vi "Execute.vi"(8 "error in":errorcluster, 11 "Stabilize Laser in":refnum<class "Stabilize Laser.lvclass">) -> (0 "error out":errorcluster, 1 "Next Step?":bool, 2 "MSG":string, 3 "Stabilize Laser out":refnum<class "Stabilize Laser.lvclass">)   [LabVIEW 2013, in "Stabilize Laser.lvclass"]
uses:
  Stabilize Laser.lvclass
  Stabilize Laser.lvclass/Stabilize Laser.ctl
  Stability Step/Stability Step.lvclass/Stability Step.ctl
  Reusable/Sequence/STEPS/STEP.lvclass/STEP.ctl
  Read State DVR.vi
  Stability Step/Read # of Obs.vi
  Reusable/Sequence/STEPS/Read First Call.vi
  Stability Step/Read Error.vi
  Reusable/Sequence/STEPS/Write First Call.vi
  Reusable/PAS/Data/Main/Read CellData.vi
  Reusable/PAS/Data/Cell/Read houseKeeping.vi
  Data/cPAS Data.lvclass
  Reusable/PAS/Data/Cell/PAS Cell Data.lvclass
  <vilib>/Analysis/NI_AALBase.lvlib
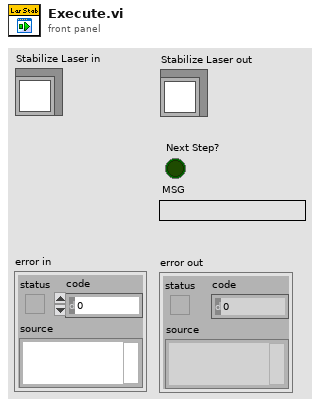
[diagram p1: front panel]
types:
  T1 = cluster{"T":sgl, "TRH":sgl, "RH":sgl, "laserRMS":sgl}
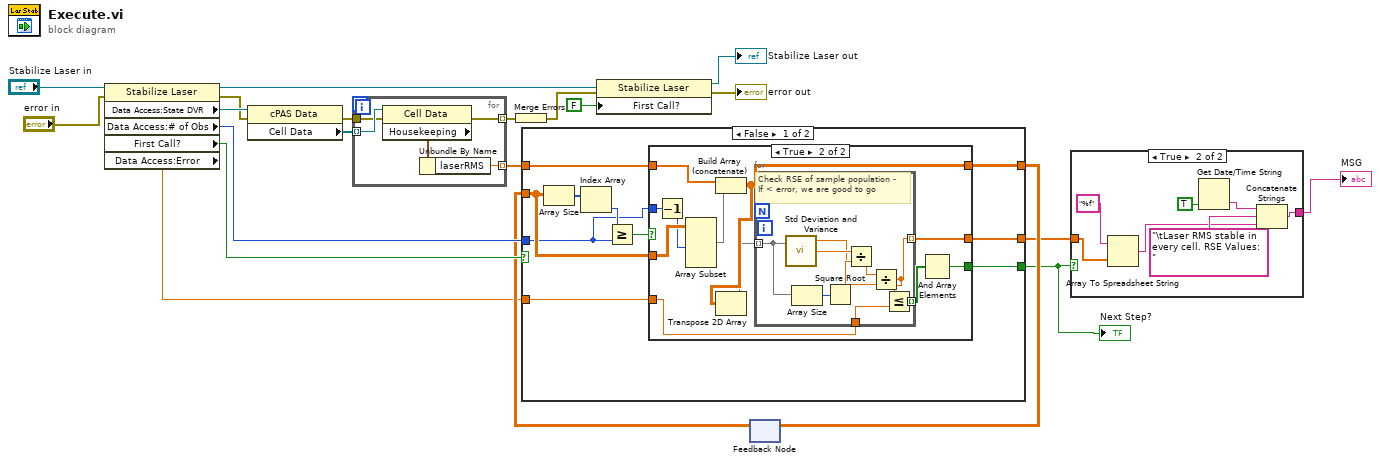
[diagram p0: block diagram]
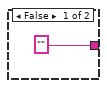
[diagram p2: hidden frame]
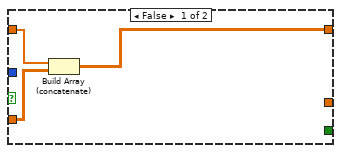
[diagram p3: hidden frame]
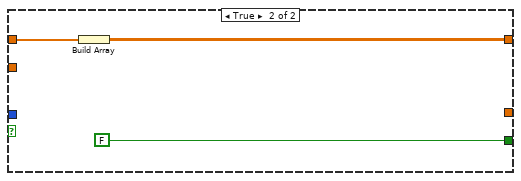
[diagram p4: hidden frame]
diagram:
  n1 = property class="Stabilize Laser"(reference="Stabilize Laser in", error in="error in") -> (reference out=w20:refnum<class "Stabilize Laser.lvclass">, error out=w3:errorcluster, "Data Access:State DVR"=w4:refnum<data-value>, "Data Access:# of Obs"=w17:u16, "First Call?"=w18:bool, "Data Access:Error"=w2:sgl)
  n2 = property class="cPAS Data"(reference=w4, error in=w3) -> (error out=w13:errorcluster, "Cell Data"=w21:refnum<class "PAS Cell Data.lvclass">[])  [unwired: 1 out]
  n3 = for {
    tunnel: w21 -> [w26] mode=indexing
    tunnel: [w24] -> w16 mode=indexing
    tunnel: w13 -> [w23]
    tunnel: [w22] -> w12 mode=indexing
    n4 = property class="Cell Data"(reference=w26, error in=w23) -> (error out=w22:errorcluster, "Housekeeping"=w25:T1)  [unwired: 1 out]
    n5 = Unbundle By Name(w25) -> ("laserRMS"=w24:sgl)
  }
  n6 = Merge Errors(w12) -> (w11:errorcluster)
  n7 = property class="Stabilize Laser"(reference=w20, error in=w11, "First Call?"=FALSE) -> (reference out=→"Stabilize Laser out":refnum<class "Stabilize Laser.lvclass">, error out=→"error out":errorcluster)
  n8 = feedback #1() -> (w14:sgl[][])  [unwired: 1 in]
  n9 = case shown="False" w18 {
    tunnel: w17 -> [w28 _]
    tunnel: w16 -> [w34 w62]
    tunnel: [w32 w61] -> w15
    tunnel: w14 -> [w33 _]
    tunnel: [w29 FALSE ("Boolean")] -> w5
    tunnel: w2 -> [w30 _]
    tunnel: [w27 _] -> w1
    frame False {
      n10 = Array Size(array=w33) -> (size(s)=w36:i32[])
      n11 = Index Array(array=w36) -> (element=w31:i32)  [unwired: 1 in]
      n12 = Greater Or Equal?(x=w31, y=w28) -> (x >= y?=w35:bool)
      n13 = case shown="True" w35 {
        tunnel: w34 -> [w39 w48]
        tunnel: w33 -> [w38 w50]
        tunnel: [w37 w44] -> w32
        tunnel: w30 -> [_ w41]
        tunnel: [_ w47] -> w29
        tunnel: w28 -> [_ w46]
        tunnel: [_ w42] -> w27
        frame False {
          n14 = Build Array (concatenate)(w39, w38) -> (w37:sgl[][])
        }
        frame True {
          n15 = Decrement(x=w46) -> (x-1=w45:u16)
          n16 = Array Subset(array=w50, length (row)=w45) -> (w49:sgl[][])  [unwired: 3 in]
          n17 = Build Array (concatenate)(w48, w49) -> (w44:sgl[][])
          n18 = Transpose 2D Array(2D array=w44) -> (transposed array=w43:sgl[][])
          n19 = for {
            tunnel: w43 -> [w59] mode=indexing
            tunnel: [w53] -> w42 mode=indexing
            tunnel: w41 -> [w52]
            tunnel: [w51] -> w40 mode=indexing
            # "Check RSE of sample population -\nIf < error, we are good to go"
            n20 = call <vilib>:"Std Deviation and Variance.vi"("X"=w59) -> ("mean"=w54:dbl, "standard deviation"=w57:dbl)  [unwired: 1 in, 1 out]
            n21 = Array Size(array=w59) -> (size(s)=w58:i32)
            n22 = Square Root(x=w58) -> (sqrt(x)=w56:dbl)
            n23 = Divide(x=w57, y=w56) -> (x/y=w55:dbl)
            n24 = Divide(x=w55, y=w54) -> (x/y=w53:dbl)
            n25 = Less Or Equal?(x=w53, y=w52) -> (x <= y?=w51:bool)
          }
          n26 = And Array Elements(Boolean array=w40) -> (logical AND=w47:bool)
        }
      }
    }
    frame True {
      n27 = Build Array(w62) -> (w61:sgl[][])
    }
  }
  "Next Step?" <- w5
  n28 = feedback-in #1(w15) -> ()
  n29 = case shown="True" w5 {
    tunnel: ["" w68] -> w6
    tunnel: w1 -> [_ w64]
    frame False {
    }
    frame True {
      n30 = Array To Spreadsheet String(array=w64, 3:"%f" ("format string")) -> (spreadsheet string=w66:string)  [unwired: 1 in]
      n31 = Get Date/Time String(want seconds? (F)=TRUE) -> (time string=w69:string)  [unwired: 2 in, 1 out]
      n32 = Concatenate Strings(w69, "\tLaser RMS stable in every cell. RSE Values: " ("string"), w66) -> (w68:string)
    }
  }
  "MSG" <- w6
